vi "Debug - TCP - Default Log Filename--Const.vi"() -> (3 "Debug Log Filename":string)   [LabVIEW 2017, in "Communications Library.lvlib"]
uses:
  Communications Library.lvlib
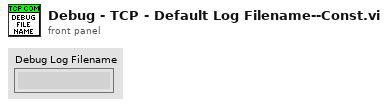
[diagram p1: front panel]
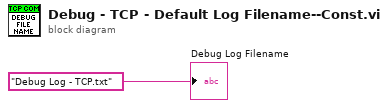
[diagram p0: block diagram]
diagram:
  "Debug Log Filename" <- "Debug Log - TCP.txt" ("data in")
